vi "Lockin-4461 IV mode trigger and wait.vi"(5 "Port":u16, 7 "address":string, 8 "error in (no error)":errorcluster, 10 "Channels: AO":T1={"AO Amp (V)"=[1.0, 0.0, 0.0, 0.0, 0.0, 0.0, 0.0, 0.0], "AO DC (V)"=[0.0, 0.0, 0.0, 0.0, 0.0, 0.0, 0.0, 0.0], "AO f (Hz)"=[1.0, 1.0, 1.0, 1.0, 1.0, 1.0, 1.0, 1.0], "AO Phase (°)"=[0.0, 0.0, 0.0, 0.0, 0.0, 0.0, 0.0, 0.0], "Function"=[enum."Triangle", enum."Sine", enum."Sine", enum."Sine", enum."Sine", enum."Sine", enum."Sine", enum."Sine"], "I+"=[], "Sweeping"=[]} {"AO f (Hz)" min=0.001 max=10000.0; "AO DC (V)" format="%.3p"; "AO Amp (V)" format="%.3p"}, 11 "Instrument.Lockin in":refnum<class "Instrument.Lockin.lvclass">) -> (0 "error out":errorcluster, 2 "input signal":waveform(dbl)[](array[waveform]), 3 "Instrument.Lockin out":refnum<class "Instrument.Lockin.lvclass">)   [LabVIEW 2016]
uses:
  Instrument.Lockin/Typedefs/AO-cluster.ctl
  Instrument.Lockin/Typedefs/AO_Amp-array.ctl
  Instrument.Lockin/Typedefs/AO_DC-array.ctl
  Instrument.Lockin/Typedefs/AO_f-array.ctl
  Instrument.Lockin/Typedefs/AO_phi-array.ctl
  Instrument.Lockin/Typedefs/Function-array.ctl
  Instrument.Lockin/Typedefs/Function-enum.ctl
  Instrument.Lockin/Instrument.Lockin.lvclass
panel:
  in  "stop":bool
  out "timer (s)":dbl=1.2239999771118164
  # "This VI triggers the lockin and waits until the acquisition is complete"
  # "1"
  # "2"
  # "3"
  # "4"
  # "5"
  # "6"
  # "7"
  # "8"
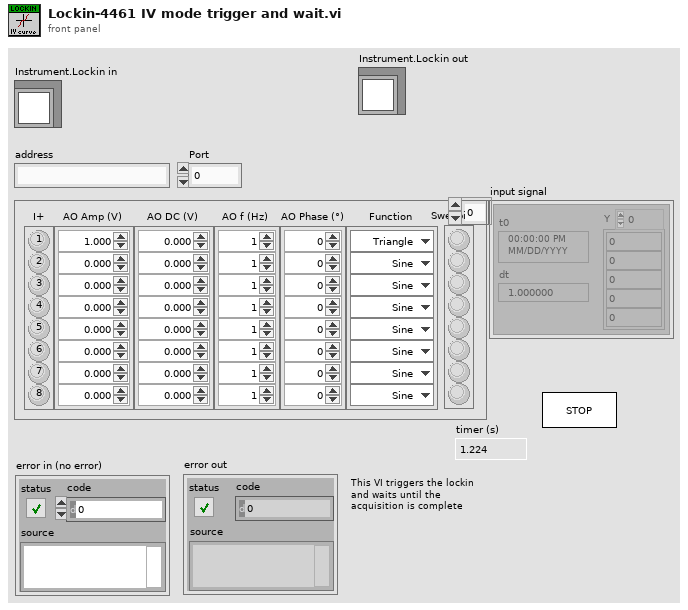
[diagram p1: front panel]
types:
  T1 = typedef "Instrument.Lockin.lvclass/AO-cluster.ctl" = cluster{"AO Amp (V)":T2, "AO DC (V)":T3, "AO f (Hz)":T4, "AO Phase (°)":T5, "Function":T6, "I+":bool[], "Sweeping":bool[]}
  T2 = typedef "Instrument.Lockin.lvclass/AO_Amp-array.ctl" = dbl[]
  T3 = typedef "Instrument.Lockin.lvclass/AO_DC-array.ctl" = dbl[]
  T4 = typedef "Instrument.Lockin.lvclass/AO_f-array.ctl" = dbl[]
  T5 = typedef "Instrument.Lockin.lvclass/AO_phi-array.ctl" = dbl[]
  T6 = typedef "Instrument.Lockin.lvclass/Function-array.ctl" = T7[]
  T7 = typedef "Instrument.Lockin.lvclass/Function-enum.ctl" = enum16{"Sine", "Triangle", "Square", "Sawtooth"}
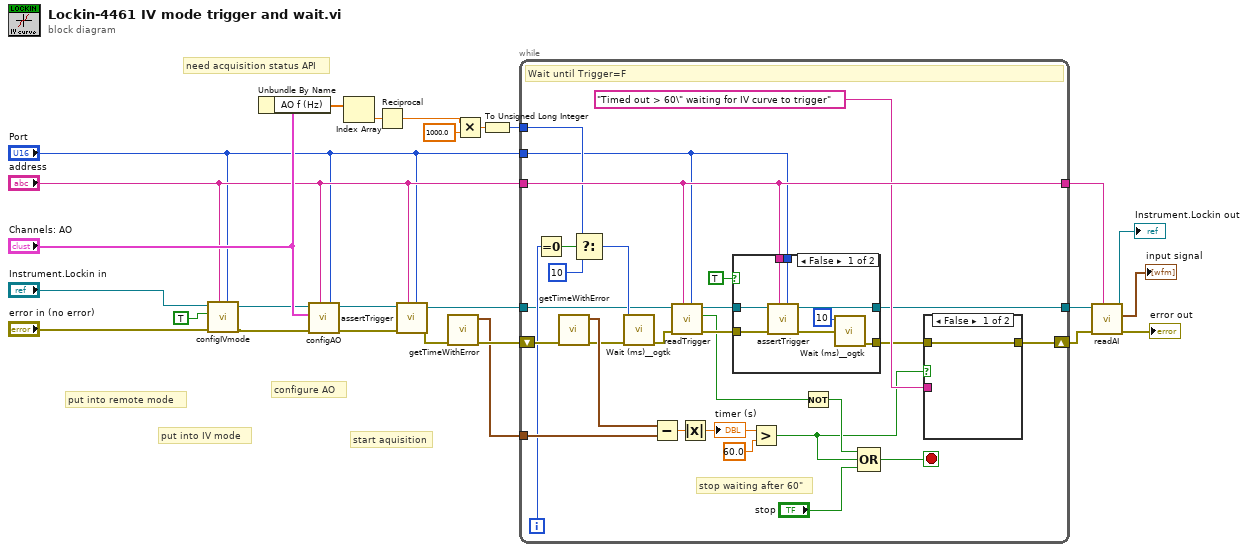
[diagram p0: block diagram]
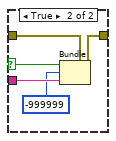
[diagram p2: hidden frame]
diagram:
  # "need acquisition status API"
  # "start aquisition"
  # "configure AO"
  # "put into IV mode"
  # "put into remote mode"
  n1 = call "configIVmode.vi"("Port"="Port", "address"="address", "error in (no error)"="error in (no error)", "IV mode"=TRUE, "Instrument.Lockin in"="Instrument.Lockin in") -> ("error out"=w25:errorcluster, "Instrument.Lockin out"=w2:refnum<class "Instrument.Lockin.lvclass">)  [unwired: 5 in]
  n2 = Unbundle By Name("Channels: AO") -> ("AO f (Hz)"=w18:T4)
  n3 = call "configAO.vi"("Port"="Port", "address"="address", "error in (no error)"=w25, "Channels: AO in"="Channels: AO", "Instrument.Lockin in"=w2) -> ("error out"=w24:errorcluster, "Instrument.Lockin out"=w3:refnum<class "Instrument.Lockin.lvclass">)  [unwired: 5 in]
  n4 = Index Array(array=w18) -> (element=w17:dbl)  [unwired: 1 in]
  n5 = Reciprocal(x=w17) -> (1/x=w14:dbl)
  n6 = call "assertTrigger.vi"("Port"="Port", "address"="address", "error in (no error)"=w24, "Instrument.Lockin in"=w3) -> ("error out"=w23:errorcluster, "Instrument.Lockin out"=w4:refnum<class "Instrument.Lockin.lvclass">)  [unwired: 6 in]
  n7 = call "getTimeWithError.vi"("error in (no error)"=w23) -> ("error out"=w22:errorcluster, "seconds since 1Jan1904"=w21:timestamp)  [unwired: 9 in]
  n8 = Multiply(x=w14, y=1000.0) -> (x*y=w15:dbl)
  n9 = To Unsigned Long Integer(number=w15) -> (unsigned 32bit integer=w13:u32)
  n10 = while {
    tunnel: "address" -> [w45]
    shift-right: [w43] -> w20
    shift-left: w22 -> [w51]
    tunnel: [w45] -> w10
    tunnel: w21 -> [w49]
    tunnel: w13 -> [w33]
    tunnel: [w31] -> w7
    tunnel: "Port" -> [w30]
    tunnel: w4 -> [w28]
    i -> [w37]
    stop <- w47 stop-if-true
    # "stop waiting after 60\""
    # "Wait until Trigger=F"
    n11 = Equal To 0?(x=w37) -> (x = 0?=w36:bool)
    n12 = call "getTimeWithError.vi"("error in (no error)"=w51) -> ("error out"=w40:errorcluster, "seconds since 1Jan1904"=w50:timestamp)  [unwired: 9 in]
    n13 = Select(t=w33, s=w36, f=u32 10) -> (s? t:f=w34:u32)
    n14 = call <userlib>:"Wait (ms)__ogtk.vi"("error in (no error)"=w40, "milliseconds to wait"=w34) -> ("error out"=w39:errorcluster)  [unwired: 8 in, 1 out]
    n15 = Subtract(x=w50, y=w49) -> (x-y=w54:dbl)
    n16 = call "readTrigger.vi"("Port"=w30, "address"=w45, "error in (no error)"=w39, "Instrument.Lockin"=w28) -> ("error out"=w46:errorcluster, "Trigger"=w32:bool, "Instrument.Lockin"=w29:refnum<class "Instrument.Lockin.lvclass">)  [unwired: 5 in]
    n17 = Absolute Value(x=w54) -> (abs(x)=w52:dbl)
    "timer (s)" <- w52
    n18 = case shown="False" TRUE {
      tunnel: w46 -> [w68 w70]
      tunnel: w45 -> [w67 _]
      tunnel: [w64 w70] -> w27
      tunnel: [w63 w69] -> w31
      tunnel: w30 -> [w62 _]
      tunnel: w29 -> [w61 w69]
      frame False {
        n19 = call "assertTrigger.vi"("Port"=w62, "address"=w67, "error in (no error)"=w68, "Instrument.Lockin in"=w61) -> ("error out"=w65:errorcluster, "Instrument.Lockin out"=w63:refnum<class "Instrument.Lockin.lvclass">)  [unwired: 6 in]
        n20 = call <userlib>:"Wait (ms)__ogtk.vi"("error in (no error)"=w65, "milliseconds to wait"=u32 10) -> ("error out"=w64:errorcluster)  [unwired: 8 in, 1 out]
      }
      frame True {
      }
    }
    n21 = Greater?(x=w52, y=60.0) -> (0:w41:bool)
    n22 = Not(x=w32) -> (.not. x?=w48:bool)
    n23 = Compound Arithmetic op=OR(w48, w41, "stop") -> (w47:bool)
    n24 = case shown="False" w41 {
      selector: w41 -> [_ w58]
      tunnel: "Timed out > 60\" waiting for IV curve to trigger" ("source") -> [_ w60]
      tunnel: w27 -> [w55 w59]
      tunnel: [w55 w57] -> w43
      frame False {
      }
      frame True {
        n25 = Bundle(cluster=w59, "status"=w58, "code"=-999999, "source"=w60) -> (w57:errorcluster)
      }
    }
  }
  n26 = call "readAI.vi"("address"=w10, "error in (no error)"=w20, "Instrument.Lockin in"=w7) -> ("error out"=→"error out":errorcluster, "input signal"=→"input signal":waveform(dbl)[], "Instrument.Lockin out"=→"Instrument.Lockin out":refnum<class "Instrument.Lockin.lvclass">)  [unwired: 6 in]
